vi "testParseStateQueueCheckEventsHandling.vi"(8 "error in (no error)":errorcluster, 11 "testStateMachineUtilities in":refnum<class "testStateMachineUtilities.lvclass">) -> (0 "error out":errorcluster, 3 "testStateMachineUtilities out":refnum<class "testStateMachineUtilities.lvclass">)   [LabVIEW 2013, in "testStateMachineUtilities.lvclass"]
uses:
  testStateMachineUtilities.lvclass
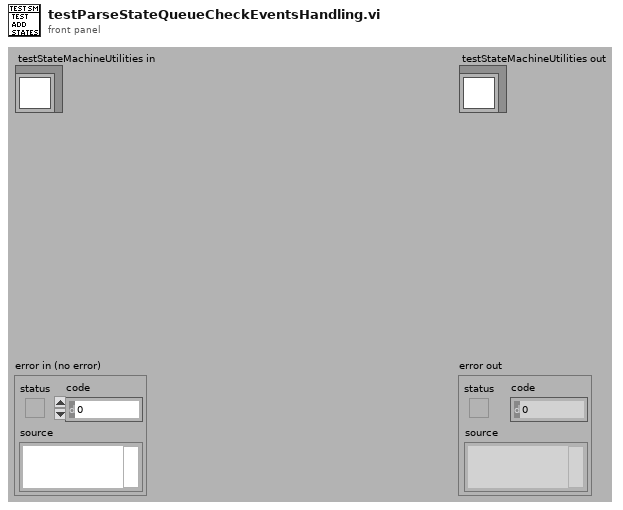
[diagram p1: front panel]
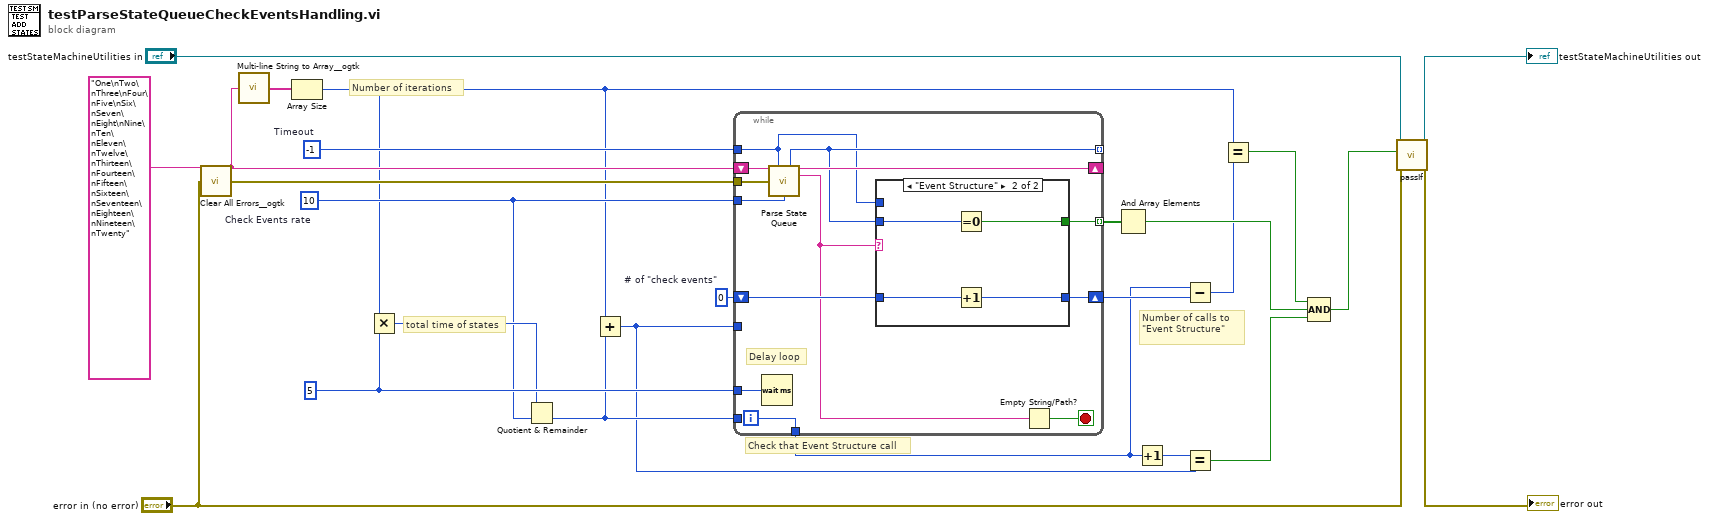
[diagram p0: block diagram]
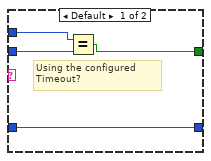
[diagram p2: hidden frame]
diagram:
  w12 = 0  # # of "check events"
  w11 = u32 5 ("milliseconds to wait")
  w9 = 10  # Check Events rate
  w17 = -1  # Timeout
  w19 = "One\nTwo\nThree\nFour\nFive\nSix\nSeven\nEight\nNine\nTen\nEleven\nTwelve\nThirteen\nFourteen\nFifteen\nSixteen\nSeventeen\nEighteen\nNineteen\nTwenty" ("State Queue")
  # "total time of states"
  # "Number of iterations"
  # "Number of calls to \"Event Structure\""
  # "Check that Event Structure call"
  n1 = call <userlib>:"Clear All Errors__ogtk.vi"("Error In"="error in (no error)") -> ("Error Out"=w20:errorcluster)  [unwired: 3 in]
  n2 = call <userlib>:"Multi-line String to Array__ogtk.vi"("string"=w19) -> ("lines"=w18:string[])
  n3 = Array Size(array=w18) -> (size(s)=w3:i32)
  n4 = Multiply(x=w3, y=w11) -> (x*y=w10:u32)
  n5 = Quotient & Remainder(x=w10, y=w9) -> (floor(x/y)=w8:u32)  [unwired: 1 out]
  n6 = Add(x=w3, y=w8) -> (x+y=w7:u32)
  n7 = while {
    tunnel: w20 -> [w36]
    shift-right: [w35] -> _
    shift-left: w19 -> [w37]
    tunnel: w17 -> [w30]
    tunnel: [w32] -> _ mode=indexing
    tunnel: w9 -> [w34]
    tunnel: w11 -> [w33]
    tunnel: [w31] -> w16 mode=indexing
    shift-right: [w29] -> w5
    shift-left: w12 -> [w28]
    tunnel: w8 -> [_]
    tunnel: w7 -> [_]
    tunnel: [w25] -> w2
    i -> [w25]
    stop <- w27 stop-if-true
    # "Delay loop"
    n8 = Wait (ms)(milliseconds to wait=w33) -> ()  [unwired: 1 out]
    n9 = call "Parse State Queue.vi"("State Queue"=w37, "Timeout"=w30, "Check Events rate"=w34, "Error In (no error)"=w36) -> ("Timeout out"=w32:i32, "Remaining States"=w35:string, "Current State"=w26:string)  [unwired: 8 in, 1 out]
    n10 = case shown="\"Event Structure\"" w26 {
      tunnel: w32 -> [w41 w45]
      tunnel: [w39 w44] -> w31
      tunnel: w30 -> [w40 _]
      tunnel: [w38 w42] -> w29
      tunnel: w28 -> [w38 w43]
      frame Default {
        # "Using the configured Timeout?"
        n11 = Equal?(x=w40, y=w41) -> (x = y?=w39:bool)
      }
      frame "Event Structure" {
        n12 = Equal To 0?(x=w45) -> (x = 0?=w44:bool)
        n13 = Increment(x=w43) -> (x+1=w42:i32)
      }
    }
    n14 = Empty String/Path?(string/path=w26) -> (empty?=w27:bool)
  }
  n15 = And Array Elements(Boolean array=w16) -> (logical AND=w15:bool)
  n16 = Increment(x=w2) -> (x+1=w6:i32)
  n17 = Subtract(x=w2, y=w5) -> (x-y=w4:i32)
  n18 = Equal?(x=w6, y=w7) -> (x = y?=w14:bool)
  n19 = Equal?(x=w3, y=w4) -> (x = y?=w1:bool)
  n20 = Compound Arithmetic op=AND(w1, w15, w14) -> (w13:bool)
  n21 = call-dynamic "passIf.vi"("error in (no error)"="error in (no error)", "pass"=w13, "TestCase in"="testStateMachineUtilities in") -> ("error out"=→"error out":errorcluster, "TestCase out"=→"testStateMachineUtilities out":refnum<class "testStateMachineUtilities.lvclass">)  [unwired: 7 in]
